vi "Accumulcate Execution Time.vi"(10 "Result":T1={"Name"="", "Message"="", "Description"="", "Status"=enum."Passed", "Result Type"=enum."Case", "Execution Time"=0.0}, 11 "Result Model in":refnum<class "Result Model.lvclass">) -> (3 "Result Model out":refnum<class "Result Model.lvclass">)   [LabVIEW 2020, in "Result Model.lvclass"]
uses:
  Result Model.lvclass
  Core/Result/Result.ctl
  Core/Result/Status.ctl
  Core/Result/Type.ctl
  Result Model.lvclass/Result Model.ctl
  <vilib>/Utility/miscctls.llb/LVMapReplaceAction.ctl
  Core/Utilities/LUnit Utilities.lvlib
  Core/Result/Result.lvlib
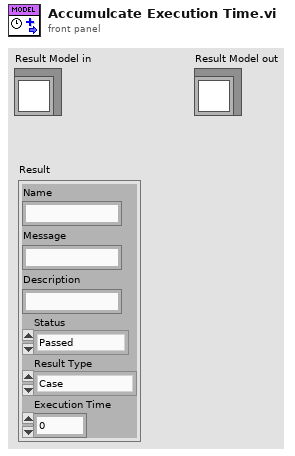
[diagram p1: front panel]
types:
  T1 = typedef "Result.lvlib/Result.ctl" = cluster{"Name":string, "Message":string, "Description":string, "Status":T2, "Result Type":T3, "Execution Time":dbl}
  T2 = typedef "Result.lvlib/Status.ctl" = enum16{"", "Passed", "Failed", "Error", "Skipped", "Setup Error", "Broken", "Teardown Error"}
  T3 = typedef "Result.lvlib/Type.ctl" = enum16{"Method", "Case", "Suite", "Pass", "Fail", "Skip", "Pass if", "Fail if", "Pass if Error", "Fail if Error", "Pass if Equal", "Fail if Equal"}
  T4 = typedef "LVMapReplaceAction.ctl" = enum32{"Modify Entry only if found", "Add or Modify Entry", "Delete Entry"}
  T5 = typedef "Result Model.lvclass/Model State.ctl" = cluster{"Run Queue":set{string}, "Test Statuses":map{string, T2}, "Execution Time":map{string, dbl}, "Assertions":map{string, cluster{"Result Type":T3, "Status":T2, "Message":string, "Description":string}[]}}
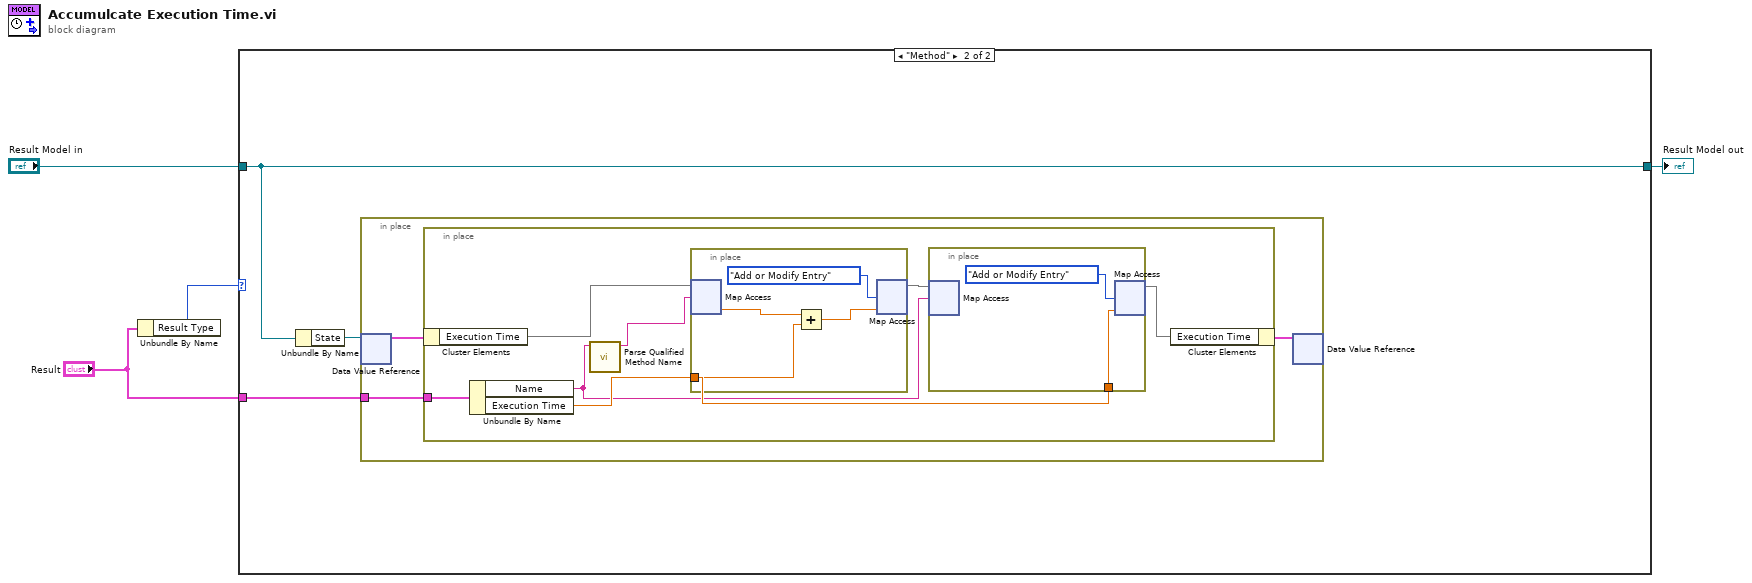
[diagram p0: block diagram]
diagram:
  n1 = Unbundle By Name("Result") -> ("Result Type"=w1:T3)
  n2 = case shown="\"Method\"" w1 {
    tunnel: "Result" -> [_ w8]
    tunnel: "Result Model in" -> [w5 w7]
    tunnel: [w5 w7] -> w3
    frame Default {
    }
    frame "Method" {
      n3 = Unbundle By Name(w7) -> ("State"=w6:refnum<data-value>)
      n4 = in-place {
        in-place-border: w8 -> [w11]
        n5 = in-place-dvr #1(w6) -> (w10:T5)  [unwired: 1 out]
        n6 = in-place {
          in-place-border: w11 -> [w17]
          n7 = in-place-cluster #2(w10) -> ("Execution Time"=w13:map{string, dbl})
          n8 = Unbundle By Name(w17) -> ("Name"=w15:string, "Execution Time"=w16:dbl)
          n9 = call "Parse Qualified Method Name.vi"("Case"=w15) -> ("Test Case Class Name"=w14:string)  [unwired: 9 in, 1 out]
          n10 = in-place {
            in-place-border: w16 -> [w22]
            n11 = in-place-map #3(w13, w14) -> (w21:dbl)  [unwired: 1 in, 1 out]
            n12 = Add(x=w21, y=w22) -> (x+y=w24:dbl)
            n13 = in-place-map #3(w24, LVMapReplaceAction."Add or Modify Entry" ("action")) -> (w18:map{string, dbl})  [unwired: 2 out]
          }
          n14 = in-place {
            in-place-border: w16 -> [w19]
            n15 = in-place-map #4(w18, w15) -> ()  [unwired: 1 in, 2 out]
            n16 = in-place-map #4(w19, LVMapReplaceAction."Add or Modify Entry" ("action")) -> (w12:map{string, dbl})  [unwired: 2 out]
          }
          n17 = in-place-cluster #2("Execution Time"=w12) -> (w9:T5)
        }
        n18 = in-place-dvr #1(w9) -> ()  [unwired: 2 out]
      }
    }
  }
  "Result Model out" <- w3
